vi "add select channel(SubVI).vi"(10 "字符串":string) -> (1 "连接的字符串":string, 2 "ok or cancel":bool=TRUE)   [LabVIEW 2019, in "Add Seq.lvlib"]
uses:
  Add Seq.lvlib
panel:
  in  "ok":bool
  in  "cancel":bool
  in  "ch2 current (mA)":dbl
  in  "ch1 current (mA)":dbl
  in  "ch2":bool
  in  "ch1":bool=TRUE
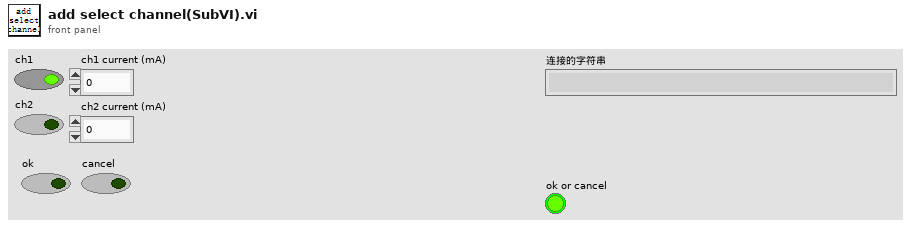
[diagram p1: front panel]
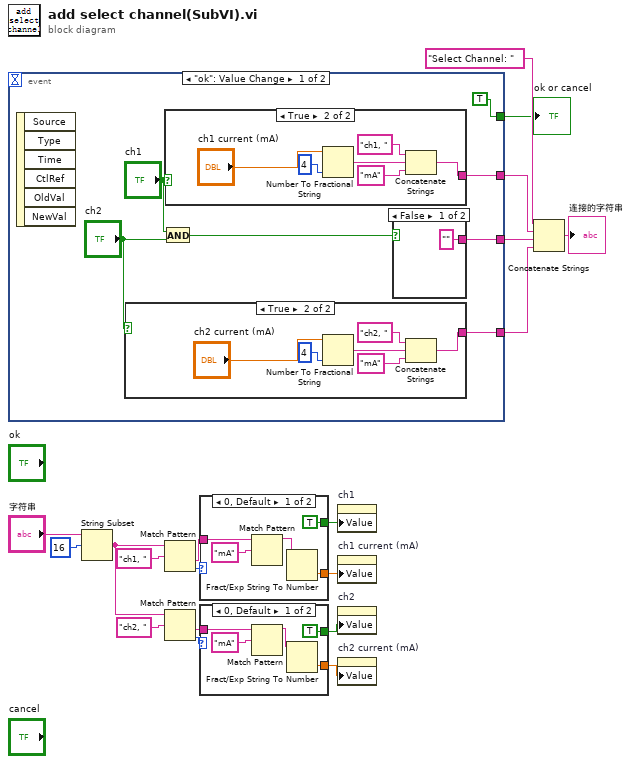
[diagram p0: block diagram]
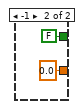
[diagram p2: hidden frame]
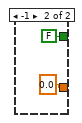
[diagram p3: hidden frame]
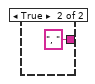
[diagram p4: hidden frame]
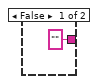
[diagram p5: hidden frame]
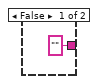
[diagram p6: hidden frame]
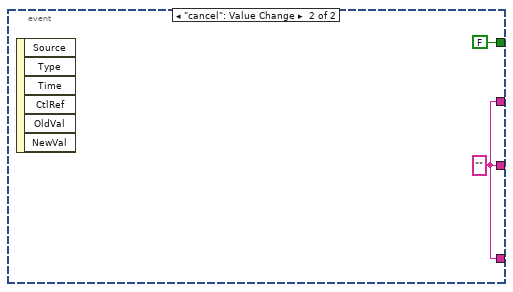
[diagram p7: hidden frame]
diagram:
  n1 = event shown="[0] \"ok\": Value Change" {
    selector: _ -> [_ _]
    dyn-events: _ -> [_ _]
    timeout: _ -> [_ _]
    tunnel: [w26 w43] -> w18
    tunnel: [w25 w43] -> w15
    tunnel: [TRUE FALSE] -> w16
    tunnel: [w20 w43] -> w14
    event "ok": Value Change {
      n2 = event-data() -> ()  [unwired: 1 in, 6 out]
      n3 = case shown="True" "ch2" {
        tunnel: ["" w30] -> w25
        frame False {
        }
        frame True {
          n4 = Number To Fractional String(number="ch2 current (mA)", precision (6)=i16 4 ("精度(6)")) -> (F-format string=w33:string)  [unwired: 2 in]
          n5 = Concatenate Strings("ch2, " ("字符串"), w33, "mA" ("字符串")) -> (w30:string)
        }
      }
      n6 = And(x="ch1", y="ch2") -> (x .and. y?=w21:bool)
      n7 = case shown="True" "ch1" {
        tunnel: ["" w37] -> w26
        frame False {
        }
        frame True {
          n8 = Number To Fractional String(number="ch1 current (mA)", precision (6)=i16 4 ("精度(6)")) -> (F-format string=w39:string)  [unwired: 2 in]
          n9 = Concatenate Strings("ch1, " ("字符串"), w39, "mA" ("字符串")) -> (w37:string)
        }
      }
      n10 = case shown="False" w21 {
        tunnel: ["" ("字符串") ", " ("字符串")] -> w20
        frame False {
        }
        frame True {
        }
      }
    }
    event "cancel": Value Change {
      w43 = ""
      n11 = event-data() -> ()  [unwired: 1 in, 6 out]
    }
  }
  "ok or cancel" <- w16
  n12 = String Subset(string="字符串", offset (0)=16 ("偏移量(0)")) -> (substring=w10:string)  [unwired: 1 in]
  n13 = Match Pattern(string=w10, regular expression="ch1, " ("正则表达式")) -> (after substring=w4:string, offset past match=w7:i32)  [unwired: 1 in, 2 out]
  n14 = Match Pattern(string=w10, regular expression="ch2, " ("正则表达式")) -> (after substring=w3:string, offset past match=w8:i32)  [unwired: 1 in, 2 out]
  n15 = case shown="0, Default" w7 {
    tunnel: [TRUE ("ch1") FALSE ("ch1")] -> w5
    tunnel: w4 -> [w47 _]
    tunnel: [w46 0.0] -> w2
    frame 0, Default {
      n16 = Match Pattern(string=w47, regular expression="mA" ("正则表达式")) -> (before substring=w45:string)  [unwired: 1 in, 3 out]
      n17 = Fract/Exp String To Number(string=w45) -> (number=w46:dbl)  [unwired: 3 in, 1 out]
    }
    frame -1 {
    }
  }
  n18 = case shown="0, Default" w8 {
    tunnel: [TRUE ("ch2") FALSE ("ch2")] -> w6
    tunnel: w3 -> [w54 _]
    tunnel: [w52 0.0] -> w1
    frame 0, Default {
      n19 = Match Pattern(string=w54, regular expression="mA" ("正则表达式")) -> (before substring=w53:string)  [unwired: 1 in, 3 out]
      n20 = Fract/Exp String To Number(string=w53) -> (number=w52:dbl)  [unwired: 3 in, 1 out]
    }
    frame -1 {
    }
  }
  n21 = property on="ch1" class="Bool (strict)"("Value"=w5) -> ()  [unwired: 2 in, 2 out]
  n22 = property on="ch1 current (mA)" class="DigNum (strict)"("Value"=w2) -> ()  [unwired: 2 in, 2 out]
  n23 = property on="ch2" class="Bool (strict)"("Value"=w6) -> ()  [unwired: 2 in, 2 out]
  n24 = property on="ch2 current (mA)" class="DigNum (strict)"("Value"=w1) -> ()  [unwired: 2 in, 2 out]
  n25 = Concatenate Strings("Select Channel: " ("字符串"), w18, w14, w15) -> (→"连接的字符串":string)
